vi "Write DIOs RT FIFO.vi"(8 "error in (no error)":errorcluster, 10 "DIO Values":bool[](array[boolean]), 11 "DIOs RT FIFO out":refnum<k33>) -> (0 "error out":errorcluster)   [LabVIEW 2021, in "RT Main.lvlib"]
uses:
  RT Main.lvlib
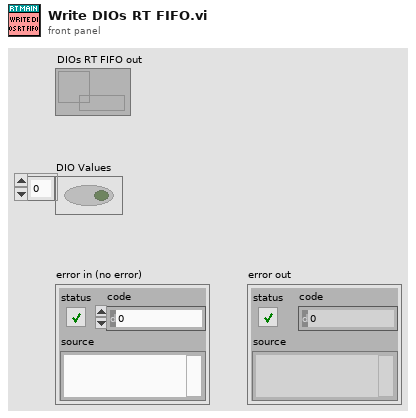
[diagram p1: front panel]
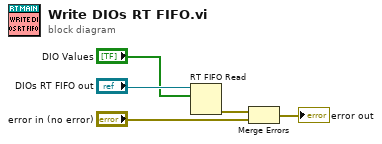
[diagram p0: block diagram]
diagram:
  n1 = RT FIFO Read(0:"DIOs RT FIFO out", 1:"DIO Values") -> (11:w3:errorcluster)  [unwired: 2 in, 4 out]
  n2 = Merge Errors(w3, "error in (no error)") -> (→"error out":errorcluster)
